vi "scan2d_close_detector.vi"(8 "error in (no error)":errorcluster, 11 "scan_2d in":refnum<class "scan_2d.lvclass">) -> (0 "error out":errorcluster, 3 "scan_2d out":refnum<class "scan_2d.lvclass">)   [LabVIEW 2015, in "scan_2d.lvclass"]
uses:
  scan_2d.lvclass
  scan_2d.lvclass/scan_2d.ctl
  Detector_Class/detector/detector.lvclass
  UI/panel_class/panel.lvclass
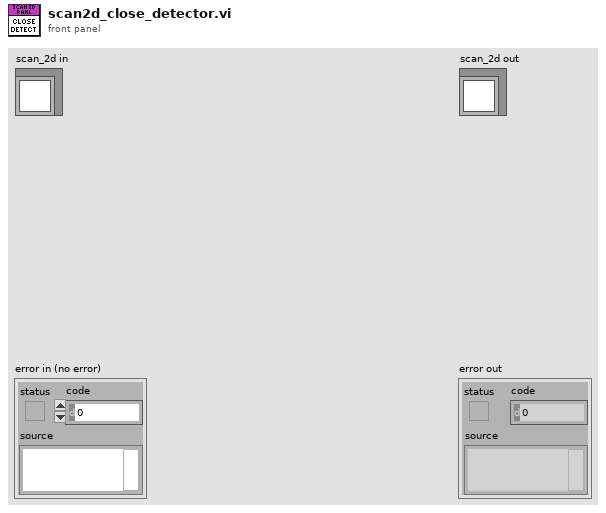
[diagram p1: front panel]
types:
  T1 = typedef "hardware_caller_queue_numbers.ctl" = enum16{"stage1", "stage2", "experiment", "detector"}
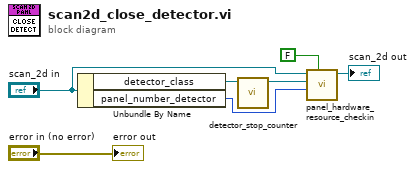
[diagram p0: block diagram]
diagram:
  n1 = Unbundle By Name("scan_2d in") -> ("detector_class"=w2:refnum<class "detector.lvclass">, "panel_number_detector"=w4:T1)
  n2 = call-dynamic "detector_stop_counter.vi"("detector in"=w2) -> ("detector out"=w1:refnum<class "detector.lvclass">)  [unwired: 9 in, 1 out]
  n3 = call "panel_hardware_resource_checkin.vi"("Self"=FALSE, "panel_number"=w4, "hardware.lvclass"=w1, "panel in"="scan_2d in") -> ("panel out"=→"scan_2d out":refnum<class "scan_2d.lvclass">)  [unwired: 6 in, 1 out]
  "error out" <- "error in (no error)"
